vi "Switch Counter Signal.vi"(5 "Incoming Page GUID":string, 6 "Invalid Count Channel GUID":string, 7 "Protected Signal GUID":string, 8 "error in (no error)":errorcluster, 9 "Signal Page GUID":string, 10 "Counter Value GUID":string, 11 "Node Ptr":T1 format="%.0x") -> (0 "error out":errorcluster)   [LabVIEW 2023, in "Protection and Counter Support System Explorer.lvlib"]
uses:
  Protection and Counter Support System Explorer.lvlib
  <vilib>/NI VeriStand/Custom Device API/Custom Device Item Ref.ctl
  <vilib>/NI VeriStand/Custom Device API/Custom Device Channel.ctl
  <vilib>/NI VeriStand/Custom Device API/Custom Device Channel Type.ctl
  <vilib>/NI VeriStand/Custom Device API/Custom Device API.lvlib
  <vilib>/NI VeriStand/Custom Device Tools/Custom Device Utility Library/Custom Device Utility Library.lvlib
  92021079-9cf3-42d0-9bb1-1c0d65f9da9b.vi
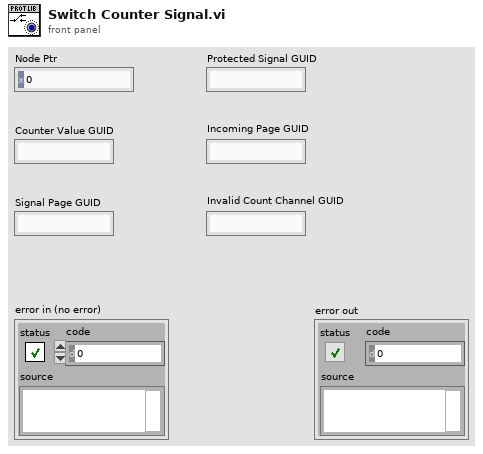
[diagram p1: front panel]
types:
  T1 = typedef "Custom Device API.lvlib/Custom Device Item Ref.ctl" = u64
  T2 = typedef "Custom Device API.lvlib/Custom Device Item Info.ctl" = cluster{"Name":string, "Is Channel":bool, "GUID":string, "Is Waveform":bool}
  T3 = typedef "Custom Device API.lvlib/Custom Device Channel.ctl" = cluster{"Type":T4, "Units":string, "Default Value":dbl, "Faultable":bool, "Scalable":bool}
  T4 = typedef "Custom Device API.lvlib/Custom Device Channel Type.ctl" = enum16{"Input", "Output"}
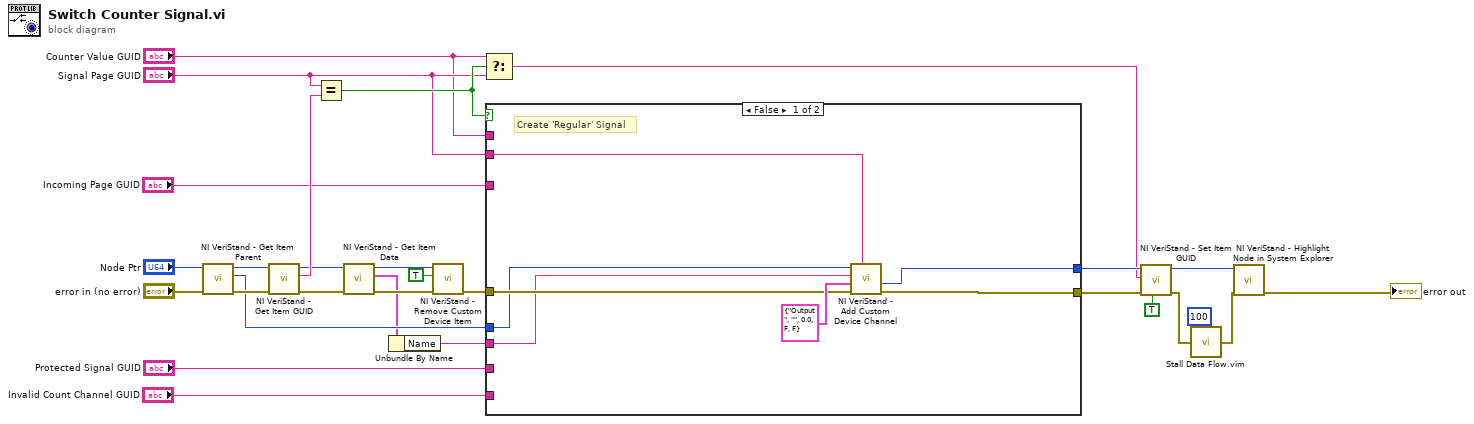
[diagram p0: block diagram]
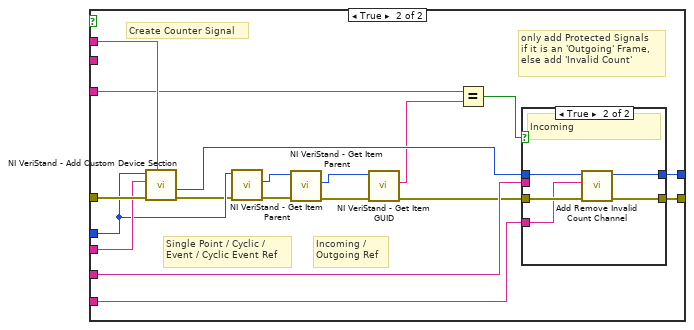
[diagram p2: hidden frame]
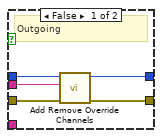
[diagram p3: hidden frame]
diagram:
  n1 = call <vilib>:"NI VeriStand - Get Item Parent.vi"("error in (no error)"="error in (no error)", "Item Ref in"="Node Ptr") -> ("error out"=w20:errorcluster, "Parent Ref"=w17:T1, "Item Ref out"=w21:T1)  [unwired: 6 in, 1 out]
  n2 = call <vilib>:"NI VeriStand - Get Item GUID.vi"("error in (no error)"=w20, "Item Ref in"=w21) -> ("error out"=w15:errorcluster, "GUID"=w24:string, "Item Ref out"=w19:T1)  [unwired: 7 in]
  n3 = Equal?(x="Signal Page GUID", y=w24) -> (x = y?=w23:bool)
  n4 = call <vilib>:"NI VeriStand - Get Item Data.vi"("error in (no error)"=w15, "Item Ref in"=w19) -> ("error out"=w14:errorcluster, "Item Info"=w13:T2, "Item Ref out"=w16:T1)  [unwired: 6 in, 1 out]
  n5 = Unbundle By Name(w13) -> ("Name"=w12:string)
  n6 = call <vilib>:"NI VeriStand - Remove Custom Device Item.vi"("error in (no error)"=w14, "Force Delete (F)"=TRUE, "Item Ref in"=w16) -> ("error out"=w18:errorcluster)  [unwired: 7 in, 1 out]
  n7 = Select(t="Counter Value GUID", s=w23, f="Signal Page GUID") -> (s? t:f=w26:string)
  n8 = case shown="False" w23 {
    tunnel: w18 -> [w35 w53]
    tunnel: [w31 w54] -> w28
    tunnel: w17 -> [w34 w47]
    tunnel: [w30 w48] -> w29
    tunnel: "Signal Page GUID" -> [w33 _]
    tunnel: w12 -> [w32 w51]
    tunnel: "Protected Signal GUID" -> [_ w49]
    tunnel: "Counter Value GUID" -> [_ w52]
    tunnel: "Invalid Count Channel GUID" -> [_ w38]
    tunnel: "Incoming Page GUID" -> [_ w37]
    frame False {
      # "Create 'Regular' Signal"
      n9 = call <vilib>:"NI VeriStand - Add Custom Device Channel.vi"("GUID (Default Channel)"=w33, "error in (no error)"=w35, "Channel"=T3 {"Type"=enum."Output", "Units"="", "Default Value"=0.0, "Faultable"=FALSE, "Scalable"=FALSE}, "Channel Name"=w32, "Parent Ref in"=w34) -> ("error out"=w31:errorcluster, "Channel Ref"=w30:T1)  [unwired: 3 in, 2 out]
    }
    frame True {
      # "Create Counter Signal"
      # "Incoming / \nOutgoing Ref"
      # "Single Point / Cyclic / \nEvent / Cyclic Event Ref"
      # "only add Protected Signals\nif it is an 'Outgoing' Frame,\nelse add 'Invalid Count'"
      n10 = call <vilib>:"NI VeriStand - Add Custom Device Section.vi"("GUID (Default Section)"=w52, "error in (no error)"=w53, "Section Name"=w51, "Parent Ref in"=w47) -> ("error out"=w41:errorcluster, "Section Ptr"=w50:T1)  [unwired: 4 in, 2 out]
      n11 = call <vilib>:"NI VeriStand - Get Item Parent.vi"("error in (no error)"=w41, "Item Ref in"=w47) -> ("error out"=w46:errorcluster, "Parent Ref"=w45:T1)  [unwired: 6 in, 2 out]
      n12 = call <vilib>:"NI VeriStand - Get Item Parent.vi"("error in (no error)"=w46, "Item Ref in"=w45) -> ("error out"=w44:errorcluster, "Parent Ref"=w43:T1)  [unwired: 6 in, 2 out]
      n13 = call <vilib>:"NI VeriStand - Get Item GUID.vi"("error in (no error)"=w44, "Item Ref in"=w43) -> ("error out"=w40:errorcluster, "GUID"=w42:string)  [unwired: 7 in, 1 out]
      n14 = Equal?(x=w37, y=w42) -> (x = y?=w39:bool)
      n15 = case shown="True" w39 {
        tunnel: [w59 w62] -> w54
        tunnel: w50 -> [w58 w64]
        tunnel: w49 -> [w57 _]
        tunnel: [w56 w61] -> w48
        tunnel: w40 -> [w55 w63]
        tunnel: w38 -> [_ w60]
        frame False {
          # "Outgoing"
          n16 = call "Add Remove Override Channels.vi"("error in (no error)"=w55, "Protected Signal GUID"=w57, "Channel Ref in"=w58) -> ("error out"=w59:errorcluster, "Channel Ref out"=w56:T1)  [unwired: 7 in]
        }
        frame True {
          # "Incoming"
          n17 = call "Add Remove Invalid Count Channel.vi"("error in (no error)"=w63, "Invalid Count Channel GUID"=w60, "Channel Ref in"=w64) -> ("error out"=w62:errorcluster, "Channel Ref out"=w61:T1)  [unwired: 7 in]
        }
      }
    }
  }
  n18 = call <vilib>:"NI VeriStand - Set Item GUID.vi"("Refresh System Explorer Tree? (F)"=TRUE, "error in (no error)"=w28, "GUID"=w26, "Item Ref in"=w29) -> ("error out"=w3:errorcluster, "Item Ref out"=w27:T1)  [unwired: 6 in]
  n19 = call "Stall Data Flow.vim"("value in"=w3, "milliseconds to wait"=u32 100) -> ("value out"=w2:errorcluster)  [unwired: 1 out]
  n20 = call <vilib>:"NI VeriStand - Highlight Node in System Explorer.vi"("error in (no error)"=w2, "Item Ref in"=w27) -> ("error out"=→"error out":errorcluster)  [unwired: 8 in, 1 out]
